vi "Delete Instrument Addon_ex.vi"() -> ()   [LabVIEW 2019]
uses:
  <vilib>/NI VeriStand/Custom Device API/Custom Device Item Ref.ctl
  Scripting API/Scripting API.lvlib
  <vilib>/NI VeriStand/Custom Device API/Custom Device API.lvlib
panel:
  out "error out":errorcluster
  in  "instrument addon refnum":T1=18446744073709551615 format="%.0x"
  in  "error in (no error)":errorcluster
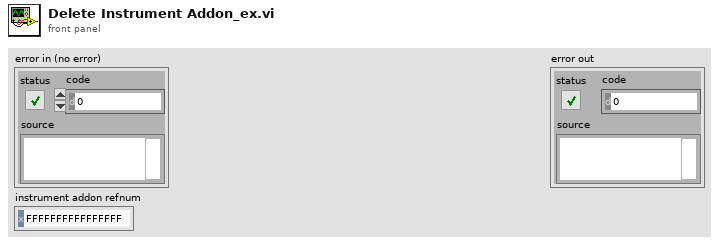
[diagram p1: front panel]
types:
  T1 = typedef "Custom Device API.lvlib/Custom Device Item Ref.ctl" = u64
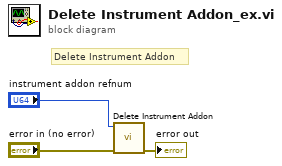
[diagram p0: block diagram]
diagram:
  # "Delete Instrument Addon"
  n1 = call "Delete Instrument Addon.vi"("error in (no error)"="error in (no error)", "instrument addon refnum"="instrument addon refnum") -> ("error out"=→"error out":errorcluster)  [unwired: 9 in]
